vi "Start Ethernet High-Speed Data Communication.vi"(0 "Device ID":i32, 1 "Max Buffer Size":u32, 7 "Ethernet Config":T1={"IP Address"=[192, 168, 0, 1], "Port No"=24692}, 9 "Start Req":T2={"High-Speed Comm Start Pos"=0, "Read Profile Cnt"=0, "High-Speed Receive Ratio"=16} {"High-Speed Receive Ratio" items=["LOWEST"=0, "LOW"=16, "MIDDLE"=17, "HIGH"=18, "HIGHEST"=32]; "High-Speed Comm Start Pos" items=["SEND COMPLETE POS", "OLDEST", "NEXT"]}, 11 "error in (no error)":errorcluster) -> (4 "Device ID out":i32, 6 "Return Code":i32, 15 "error out":errorcluster)   [LabVIEW 2014, in "Keyence LJ-V7000.lvlib"]
uses:
  Keyence LJ-V7000.lvlib
  Clusters/High-Speed Comm Start Req.ctl
  constant/High-Speed Comm Start Pos.ctl
  constant/High-Speed Receive Ratio.ctl
  Clusters/Ethernet Config.ctl
panel:
  # "(c) 2012 KEYENCE CORPORATION.  ALL RIGHTS RESERVED."
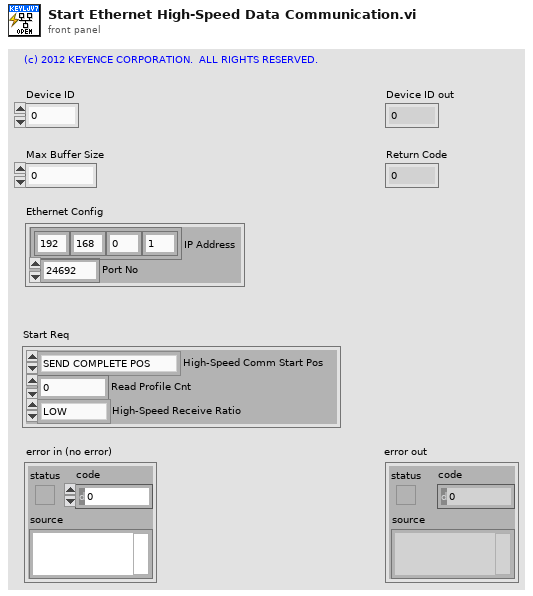
[diagram p1: front panel]
types:
  T1 = typedef "Keyence LJ-V7000.lvlib/Ethernet Config.ctl" = cluster{"IP Address":u8[], "Port No":u16}
  T2 = typedef "Keyence LJ-V7000.lvlib/High-Speed Comm Start Req.ctl" = cluster{"High-Speed Comm Start Pos":T3, "Read Profile Cnt":u32, "High-Speed Receive Ratio":T4}
  T3 = typedef "Keyence LJ-V7000.lvlib/High-Speed Comm Start Pos.ctl" = u8
  T4 = typedef "Keyence LJ-V7000.lvlib/High-Speed Receive Ratio.ctl" = u8
  T5 = cluster{"High-Speed Comm Start Pos":T3, "reserved":u8, "reserved":u8, "reserved":u8}
  T6 = cluster{"IP Address[0]":u8, "IP Address[1]":u8, "IP Address[2]":u8, "IP Address[3]":u8}
  T7 = cluster{"IP Address":cluster{"IP Address[0]":u8, "IP Address[1]":u8, "IP Address[2]":u8, "IP Address[3]":u8}, "Port No":u16, "reserved":u8, "reserved":u8}
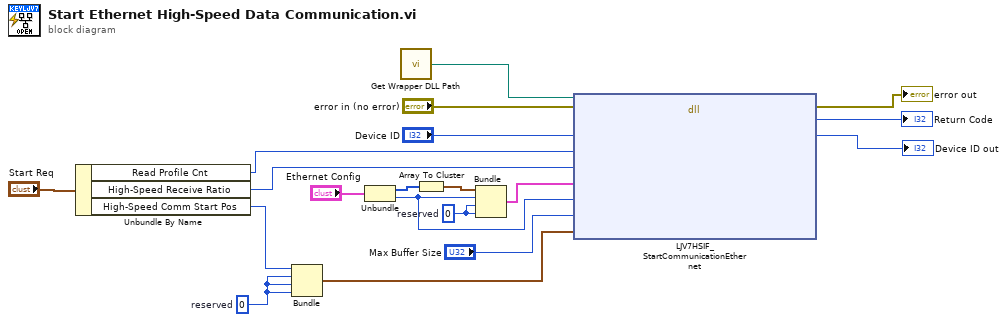
[diagram p0: block diagram]
diagram:
  w4 = u8 0  # reserved
  w9 = u8 0  # reserved
  n1 = Unbundle By Name("Start Req") -> ("Read Profile Cnt"=w12:u32, "High-Speed Receive Ratio"=w11:T4, "High-Speed Comm Start Pos"=w10:T3)
  n2 = Bundle("High-Speed Comm Start Pos"=w10, "reserved"=w9, "reserved"=w9, "reserved"=w9) -> (w8:T5)  [unwired: 1 in]
  n3 = Unbundle("Ethernet Config") -> ("IP Address"=w6:u8[], "Port No"=w1:u16)
  n4 = call "Get Wrapper DLL Path.vi"() -> ("Wrapper DLL Path"=w14:path)  [unwired: 1 in]
  n5 = Array To Cluster(array=w6) -> (cluster=w5:T6)
  n6 = Bundle("IP Address"=w5, "Port No"=w1, "reserved"=w4, "reserved"=w4) -> (w2:T7)  [unwired: 1 in]
  n7 = dll-call lib="C:/Program Files/National Instruments/LabVIEW 2011/instr.lib/Keyence LJ-V7000/LJV7_HighSpeedWrapper.dll" fn="LJV7HSIF_StartCommunicationEthernet"(path in=w14, error in="error in (no error)", "lDeviceId"="Device ID", "dwReqProfileCnt"=w12, "byReceiveRatio"=w11, "pEthernetConfig"=w2, "wHighSpeedPortNo"=w1, "dwMaxBufferSize"="Max Buffer Size", "pReq"=w8) -> (error out=→"error out":errorcluster, "lRetCode"=→"Return Code":i32, "lDeviceId"=→"Device ID out":i32)  [unwired: 7 in, 1 out]
